vi "crio_FPGA_VCA_encoder.vi"() -> ()   [LabVIEW 2019]
uses:
  <vilib>/rvi/Emulation/niFpgaSctlEmulationGetInTimedLoop.vi
  <vilib>/rvi/Emulation/niFpgaProcessEmulError.vi
  <vilib>/rvi/eio/common/nirviEmuTemplateMethod_errors.vi
  <vilib>/rvi/Emulation/niFpgaGetClockAttributes.vi
  <vilib>/rvi/Emulation/niFpgaEmulationReportErrorSimple.vi
  <vilib>/rvi/Emulation/niFpgaCriticalErrorInLSC.vi
  <vilib>/eio/EIOMethodNode/EIOMethodNode.xnode
  <vilib>/eio/EIONode/EIONode.xnode
panel:
  in  "Debug: ConnectorA/DIO15":bool
  in  "Debug: ConnectorA/DIO14":bool
  in  "Encoder Debug":bool
  in  "Loop Timer DAQ":u32=1 caption="Loop Time(uSec)"
  in  "Position Reset":bool
  out "Position (Counts)":i64
  out "B":bool
  out "A":bool
  out "B'":bool
  out "A'":bool
  in  "Velocity Interval (uSec)":u32=1000
  out "Acceleration (Counts/Interval)":i32
  out "Velocity (Counts/Interval)":i32
  in  "stop":bool
  in  "DC PWM Frequency (Hz)":sgl=20000.0
  in  "Controller PWM output [-100,100]%":sgl(slide) scale=-100.0..100.0
  out "ConnectorA/DIO13":bool
  out "ConnectorA/DIO12":bool
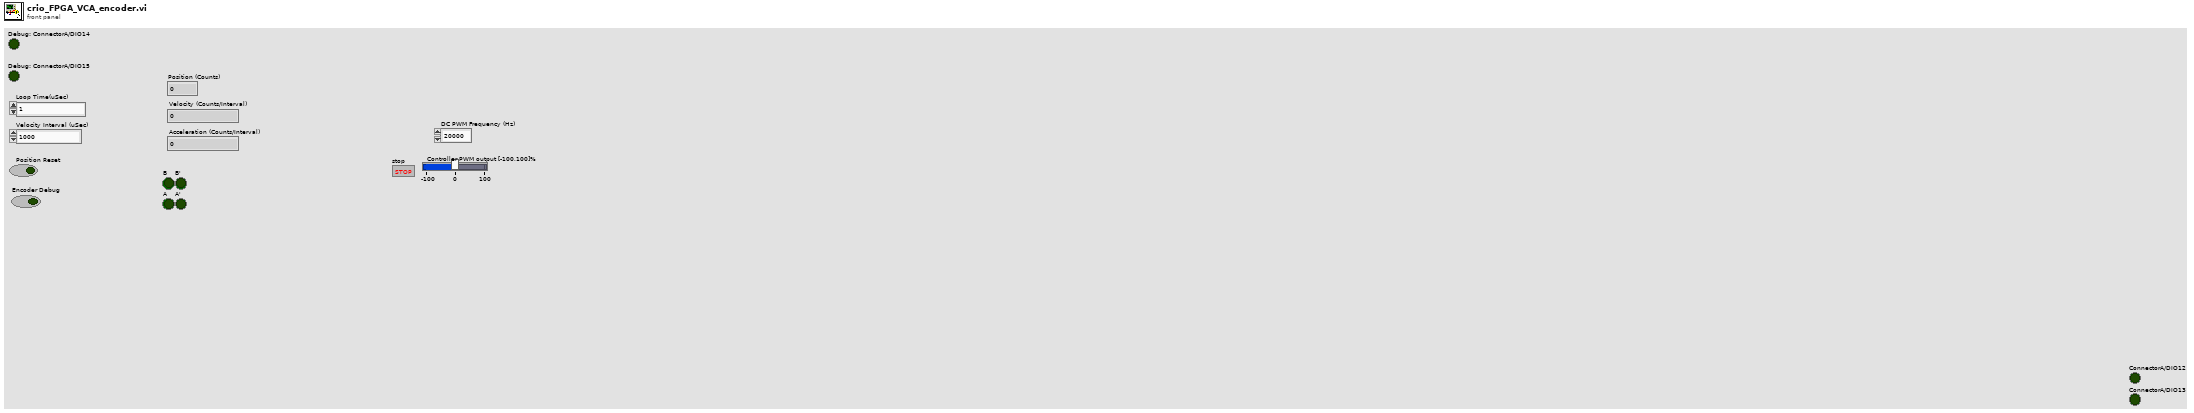
[diagram p1: front panel]
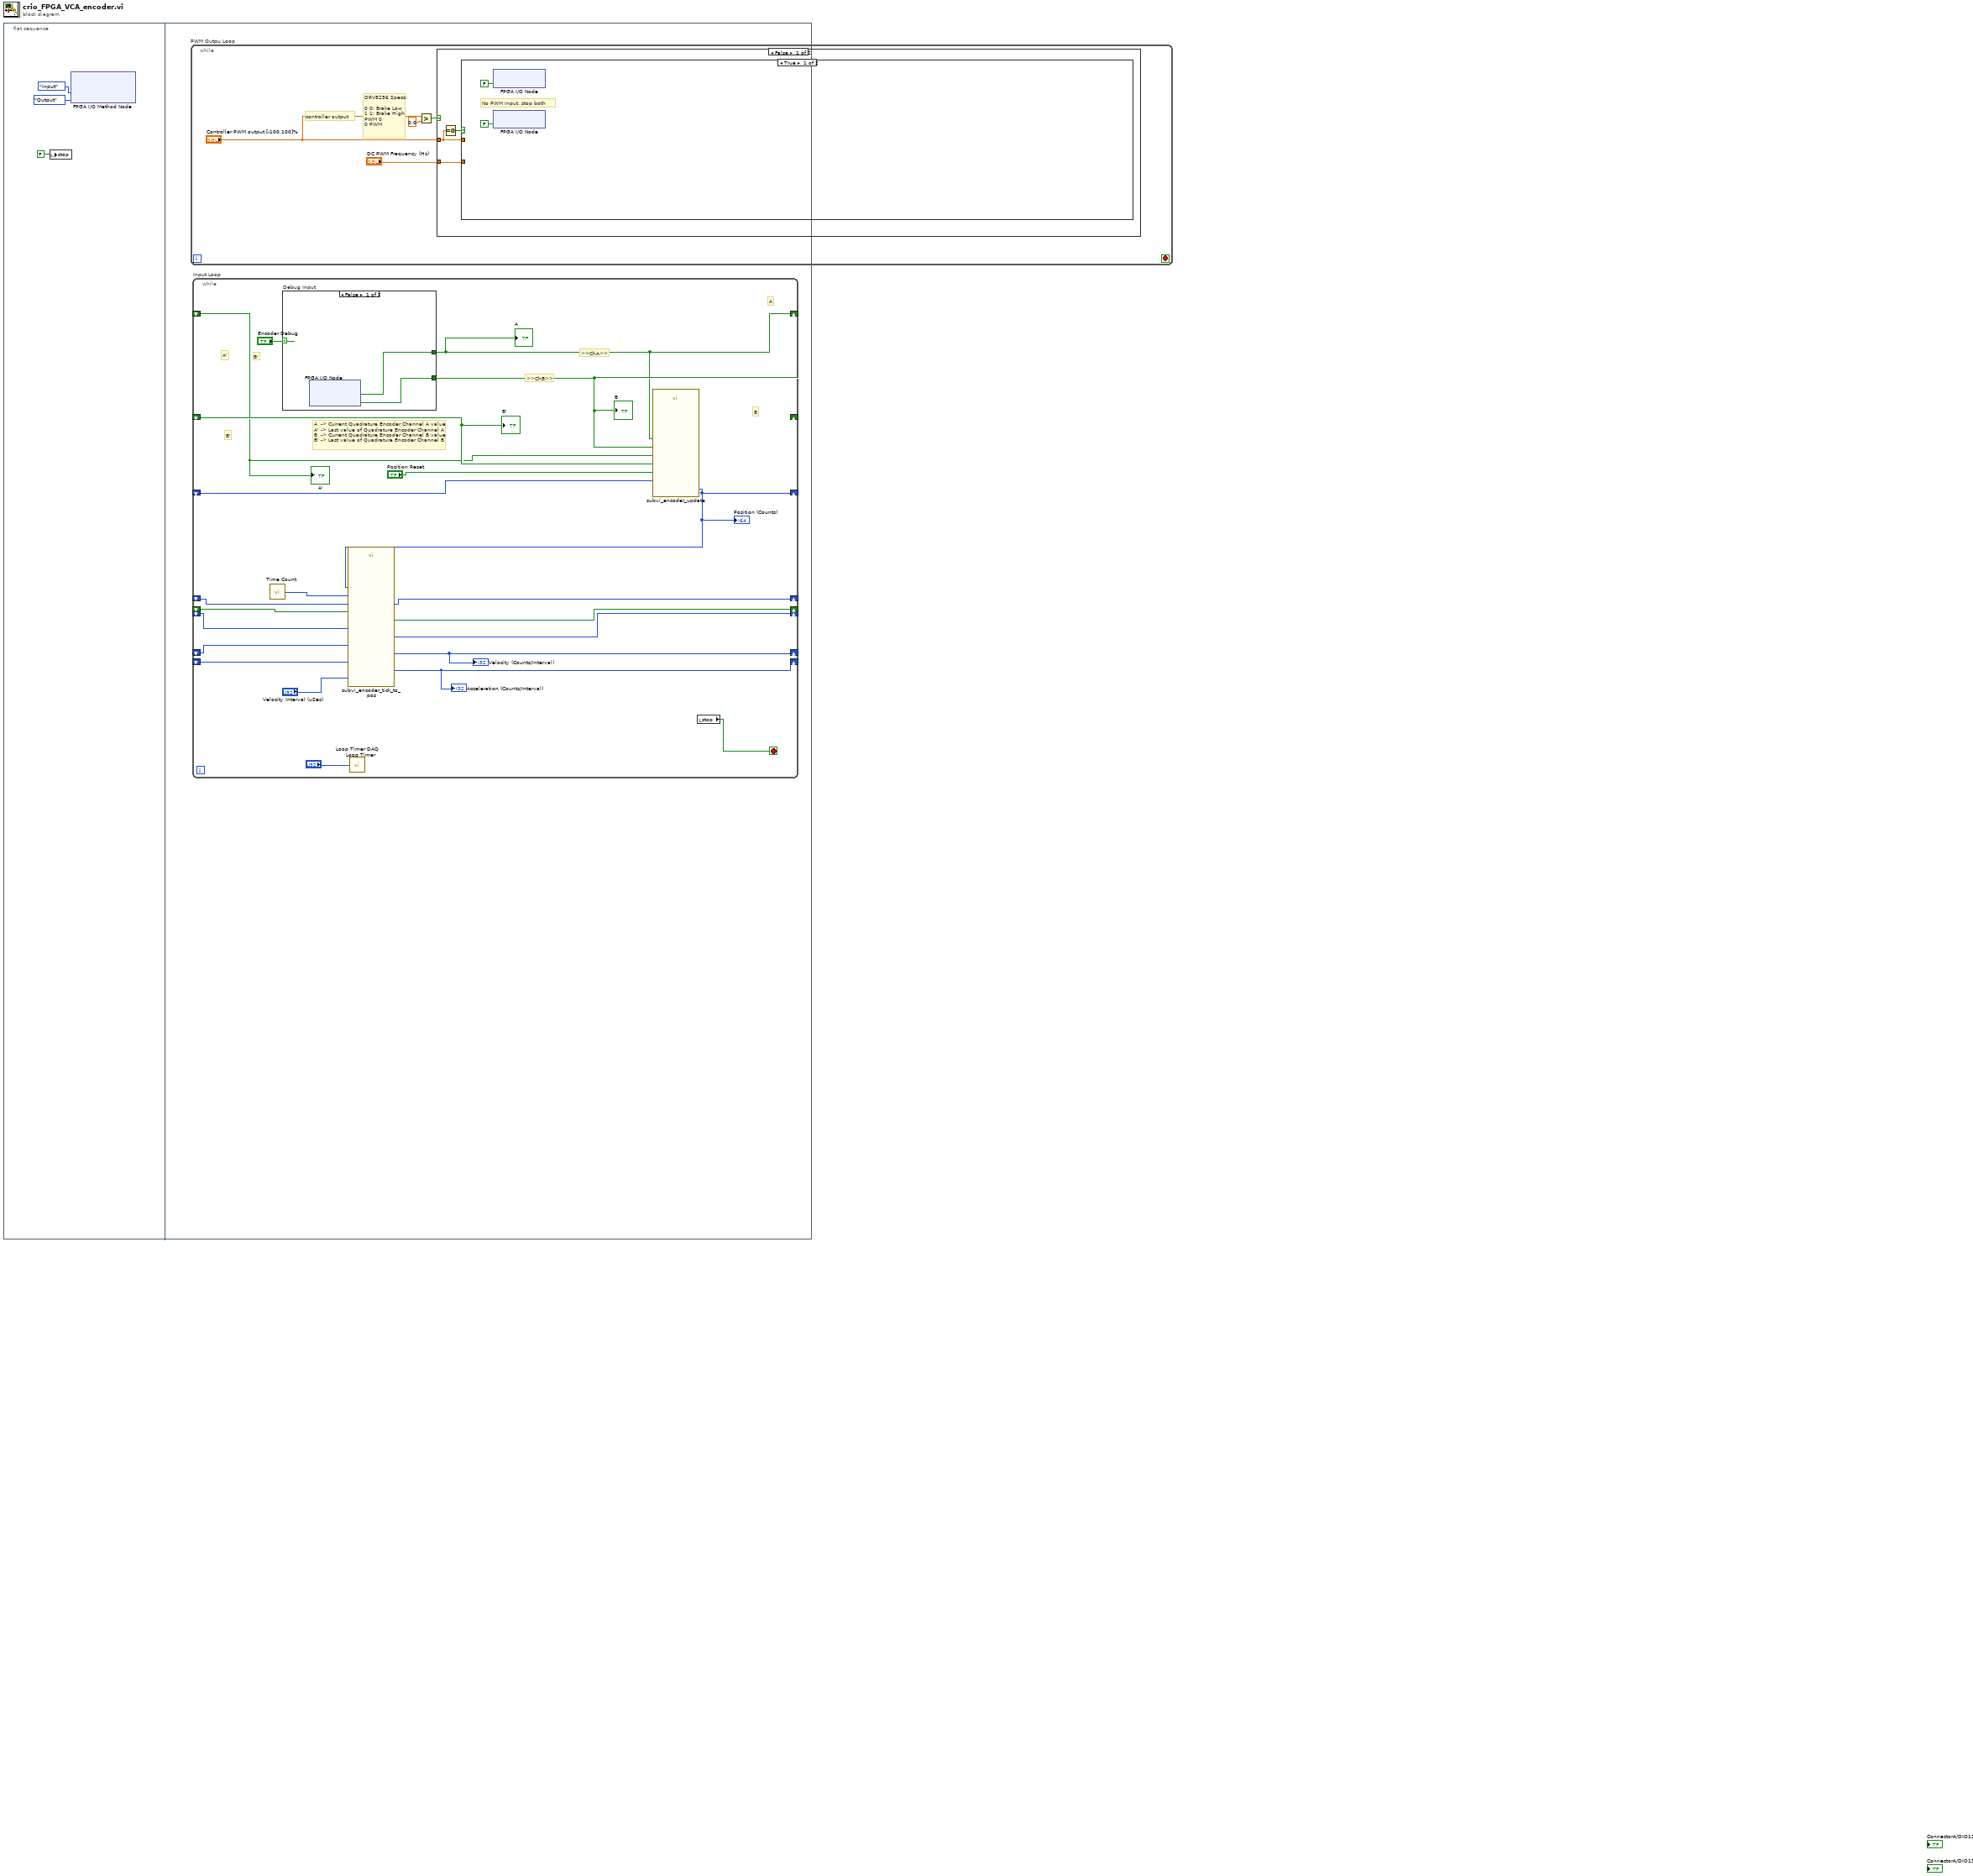
[diagram p0: block diagram]
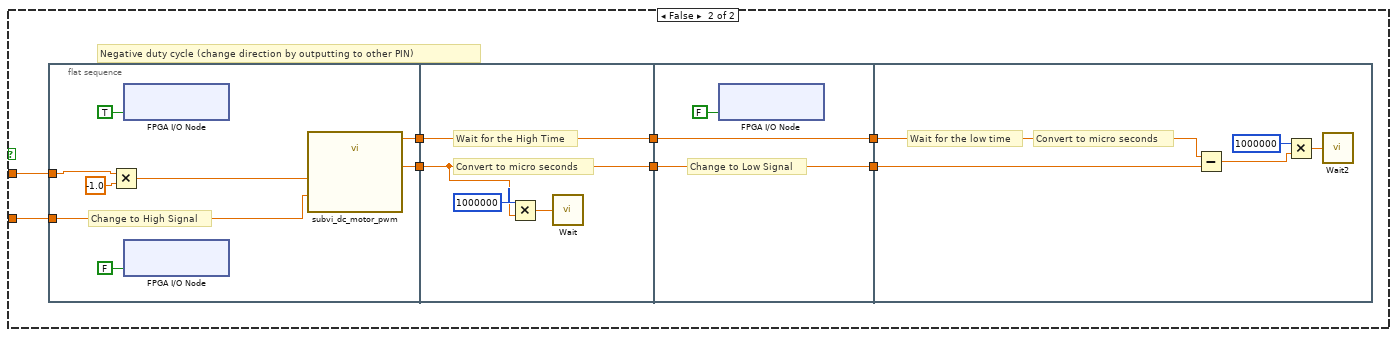
[diagram p2: hidden frame]
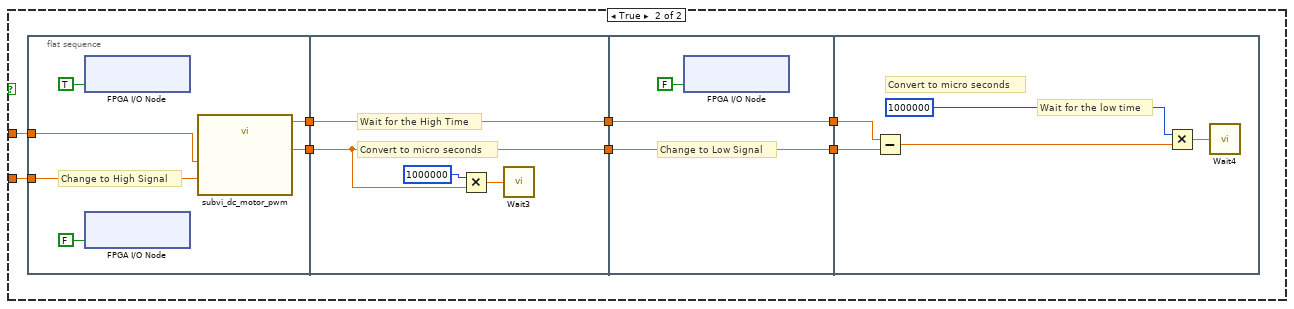
[diagram p3: hidden frame]
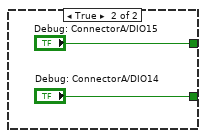
[diagram p4: hidden frame]
diagram:
  n1 = flat-sequence {
    frame #0 {
      n2 = local write "stop"(FALSE ("stop")) -> ()
      n3 = xnode "FPGA I/O Method Node"("DIO 7:4"=enum8{"No Change", "Input", "Output"}."Input", "DIO 3:0"=enum8{"No Change", "Input", "Output"}."Output") -> ()  [unwired: 1 in, 1 out]
    }
    frame #1 {
      n4 = while "PWM Outpu Loop" {
        stop <- "stop" stop-if-true
        # "DRV8256 Specs:\n\n0 0: Brake Low\n1 1: Brake High\nPWM 0\n0 PWM"
        # "controller output"
        n5 = Greater?(x="Controller PWM output [-100,100]%", y=sgl 0.0) -> (0:w5:bool)
        n6 = case shown="False" w5 {
          tunnel: "DC PWM Frequency (Hz)" -> [w11 w43]
          tunnel: "Controller PWM output [-100,100]%" -> [w10 w42]
          frame False {
            n7 = Equal To 0?(x=w10) -> (x = 0?=w9:bool)
            n8 = case shown="True" w9 {
              tunnel: w10 -> [_ w15]
              tunnel: w11 -> [_ w14]
              frame True {
                # "No PWM Input, stop both"
                n9 = xnode "FPGA I/O Node"("Mod8/DIO1"=FALSE) -> ()  [unwired: 1 in, 1 out]
                n10 = xnode "FPGA I/O Node"("Mod8/DIO0"=FALSE) -> ()  [unwired: 1 in, 1 out]
              }
              frame False {
                # "Negative duty cycle (change direction by outputting to other PIN)"
                n11 = flat-sequence {
                  tunnel: [w28] -> w21
                  tunnel: [w29] -> w20
                  tunnel: w15 -> [w25]
                  tunnel: w14 -> [w23]
                  tunnel: w21 -> [w33]
                  tunnel: [w33] -> w19
                  tunnel: w20 -> [w31]
                  tunnel: [w31] -> w18
                  tunnel: w19 -> [w35]
                  tunnel: w18 -> [w36]
                  tunnel: [w36] -> w17
                  tunnel: [w35] -> w16
                  tunnel: w17 -> [w41]
                  tunnel: w16 -> [w40]
                  frame #0 {
                    # "Change to High Signal"
                    n12 = Multiply(x=w25, y=sgl -1.0) -> (x*y=w24:sgl)
                    n13 = xnode "FPGA I/O Node"("Mod8/DIO1"=TRUE) -> ()  [unwired: 1 in, 1 out]
                    n14 = xnode "FPGA I/O Node"("Mod8/DIO0"=FALSE) -> ()  [unwired: 1 in, 1 out]
                    n15 = call "subvi_dc_motor_pwm.vi"("Duty Cycle (%)"=w24, "Frequency (Hz)"=w23) -> ("Wait time"=w29:sgl, "Cycle time"=w28:sgl)  [unwired: 8 in]
                  }
                  frame #1 {
                    # "Wait for the High Time"
                    # "Convert to micro seconds"
                    n16 = Multiply(x=u32 1000000, y=w31) -> (x*y=w30:sgl)
                    n17 = call "Wait"("Count(uSec)"=w30) -> ()  [unwired: 1 out]
                  }
                  frame #2 {
                    # "Change to Low Signal"
                    n18 = xnode "FPGA I/O Node"("Mod8/DIO1"=FALSE) -> ()  [unwired: 1 in, 1 out]
                  }
                  frame #3 {
                    # "Convert to micro seconds"
                    # "Wait for the low time"
                    n19 = Subtract(x=w40, y=w41) -> (x-y=w37:sgl)
                    n20 = Multiply(x=u32 1000000, y=w37) -> (x*y=w38:sgl)
                    n21 = call "Wait2"("Count(uSec)"=w38) -> ()  [unwired: 1 out]
                  }
                }
              }
            }
          }
          frame True {
            n22 = flat-sequence {
              tunnel: [w54] -> w49
              tunnel: [w55] -> w48
              tunnel: w43 -> [w52]
              tunnel: w42 -> [w51]
              tunnel: w49 -> [w59]
              tunnel: [w59] -> w47
              tunnel: w48 -> [w57]
              tunnel: [w57] -> w46
              tunnel: w47 -> [w61]
              tunnel: w46 -> [w62]
              tunnel: [w62] -> w45
              tunnel: [w61] -> w44
              tunnel: w45 -> [w67]
              tunnel: w44 -> [w66]
              frame #0 {
                # "Change to High Signal"
                n23 = xnode "FPGA I/O Node"("Mod8/DIO0"=TRUE) -> ()  [unwired: 1 in, 1 out]
                n24 = xnode "FPGA I/O Node"("Mod8/DIO1"=FALSE ("ConnectorB/DIO9")) -> ()  [unwired: 1 in, 1 out]
                n25 = call "subvi_dc_motor_pwm.vi"("Duty Cycle (%)"=w51, "Frequency (Hz)"=w52) -> ("Wait time"=w55:sgl, "Cycle time"=w54:sgl)  [unwired: 8 in]
              }
              frame #1 {
                # "Wait for the High Time"
                # "Convert to micro seconds"
                n26 = Multiply(x=u32 1000000, y=w57) -> (x*y=w56:sgl)
                n27 = call "Wait3"("Count(uSec)"=w56) -> ()  [unwired: 1 out]
              }
              frame #2 {
                # "Change to Low Signal"
                n28 = xnode "FPGA I/O Node"("Mod8/DIO0"=FALSE) -> ()  [unwired: 1 in, 1 out]
              }
              frame #3 {
                # "Convert to micro seconds"
                # "Wait for the low time"
                n29 = Subtract(x=w66, y=w67) -> (x-y=w63:sgl)
                n30 = Multiply(x=u32 1000000, y=w63) -> (x*y=w64:sgl)
                n31 = call "Wait4"("Count(uSec)"=w64) -> ()  [unwired: 1 out]
              }
            }
          }
        }
      }
      n32 = while "Input Loop" {
        shift-right: [w83] -> _
        shift-left: _ -> [w86]
        shift-right: [w82] -> _
        shift-left: _ -> [w85]
        shift-right: [w77] -> _
        shift-left: _ -> [w84]
        shift-right: [w69] -> _
        shift-left: _ -> [w80]
        shift-right: [w70] -> _
        shift-left: _ -> [w79]
        shift-right: [w78] -> _
        shift-left: _ -> [w76]
        shift-right: [w75] -> _
        shift-left: _ -> [w74]
        shift-right: [w73] -> _
        shift-left: _ -> [w72]
        stop <- w68 stop-if-true
        # "B'"
        # ">>ChB>>"
        # ">>ChA>>"
        # "A'"
        # "A  -> Current Quadrature Encoder Channel A value\nA' -> Last value of Quadrature Encoder Channel A\nB  -> Current Quadrature Encoder Channel B value\nB' -> Last value of Quadrature Encoder Channel B"
        # "B'"
        # "B"
        # "A"
        n33 = call "Time Count"() -> ("Tick Count(uSec)"=w71:u32)
        n34 = case "Debug Input" shown="False" "Encoder Debug" {
          tunnel: [w91 "Debug: ConnectorA/DIO15"] -> w82
          tunnel: [w90 "Debug: ConnectorA/DIO14"] -> w83
          frame False {
            n35 = xnode "FPGA I/O Node"() -> ("Mod1/DIO4"=w91:bool, "Mod1/DIO5"=w90:bool)  [unwired: 2 in, 2 out]
          }
          frame True {
          }
        }
        "B" <- w83
        "A" <- w82
        n36 = call "Loop Timer"("Count(uSec)"="Loop Timer DAQ") -> ()  [unwired: 1 out]
        n37 = call "subvi_encoder_update.vi"("Position Reset"="Position Reset", "Tick'"=w84, "A"=w82, "B'"=w86, "A'"=w85, "B"=w83) -> ("Tick"=w77:i32)  [unwired: 5 in]
        "Position (Counts)" <- w77
        n38 = call "subvi_encoder_tick_to_pos.vi"("Velocity Interval (uSec)"="Velocity Interval (uSec)", "Raw Tick"=w77, "Waited?'"=w74, "Tick Count(uSec)'"=w72, "p'"=w76, "Time Count"=w71, "a'"=w79, "v'"=w80) -> ("Waited?"=w75:bool, "Tick Count(uSec)"=w73:u32, "p"=w78:i32, "a"=w70:i32, "v"=w69:i32)  [unwired: 3 in]
        "Acceleration (Counts/Interval)" <- w70
        "Velocity (Counts/Interval)" <- w69
        n39 = local read "stop"() -> (w68:bool)
        "B'" <- w86
        "A'" <- w85
      }
    }
  }
